vi "[GV]_ALIVE.vi"() -> ()   [LabVIEW 2016]
panel:
  in  "ALIVE":u16
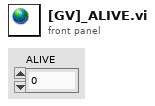
[diagram p1: front panel]
diagram:
